vi "Sub Initialize.vi"(8 "error in (no error)":errorcluster, 11 "Timer in":refnum<class "Timer.lvclass">) -> (0 "error out":errorcluster, 2 "Initialize Result":refnum<class "Acquired Result.lvclass">, 3 "Timer out":refnum<class "Timer.lvclass">)   [LabVIEW 2016, in "Timer.lvclass"]
uses:
  Timer.lvclass
  NHMFL_Core/Libraries/Instruments/Results/Acquired Result/Acquired Result.lvclass
  Timer.lvclass/Timer.ctl
  NHMFL_Core/Libraries/Instruments/Results/Acquired Result/Acquired Result.lvclass/Acquired Result.ctl
  Write Start time.vi
  Write First call.vi
  Write Delay active.vi
  NHMFL_Core/Libraries/Instruments/Results/Acquired Result/Write Channels.vi
  NHMFL_Core/Libraries/Instruments/Results/Acquired Result/Write Group.vi
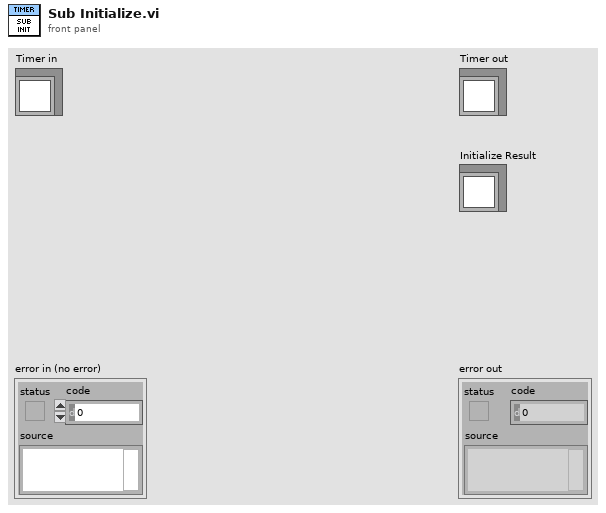
[diagram p1: front panel]
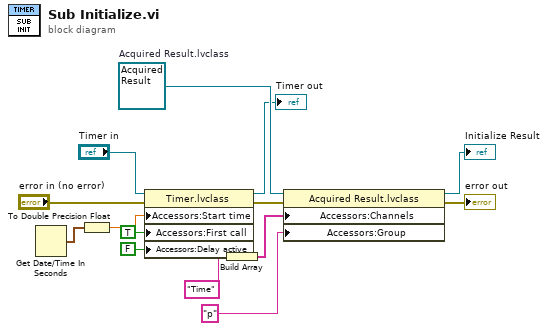
[diagram p0: block diagram]
diagram:
  w13 = refnum<class "Acquired Result.lvclass"> refnum  # Acquired Result.lvclass
  n1 = Get Date/Time In Seconds() -> (seconds since 1Jan1904=w14:timestamp)
  n2 = To Double Precision Float(number=w14) -> (double precision float=w9:dbl)
  n3 = property class="Timer.lvclass"(reference="Timer in", error in="error in (no error)", "Accessors:Start time"=w9, "Accessors:First call"=TRUE ("First call"), "Accessors:Delay active"=FALSE ("Delay active")) -> (reference out=→"Timer out":refnum<class "Timer.lvclass">, error out=w10:errorcluster)
  n4 = Build Array("Time") -> (w12:string[])
  n5 = property class="Acquired Result.lvclass"(reference=w13, error in=w10, "Accessors:Channels"=w12, "Accessors:Group"="p" ("Group")) -> (reference out=→"Initialize Result":refnum<class "Acquired Result.lvclass">, error out=→"error out":errorcluster)
